vi "Select Ch if asked and Get LR700.vi"(7 "Seconds between samples":dbl=1.0 format="%_4f", 8 "error in (no error)":errorcluster, 10 "Channels to scan (empty - don't use scanner option)":i32[](array[numeric]), 11 "VISA Resource Name":refnum<visa-resource-name>) -> (0 "error out":errorcluster, 2 "Data":dbl[](array[numeric]), 3 "VISA resource name out":refnum<visa-resource-name>)   [LabVIEW 2015]
uses:
  Get LR700 R & X_VISA.vi
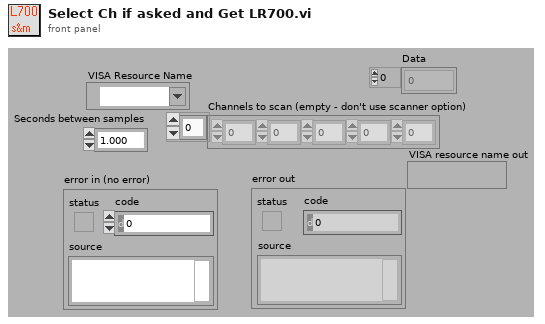
[diagram p1: front panel]
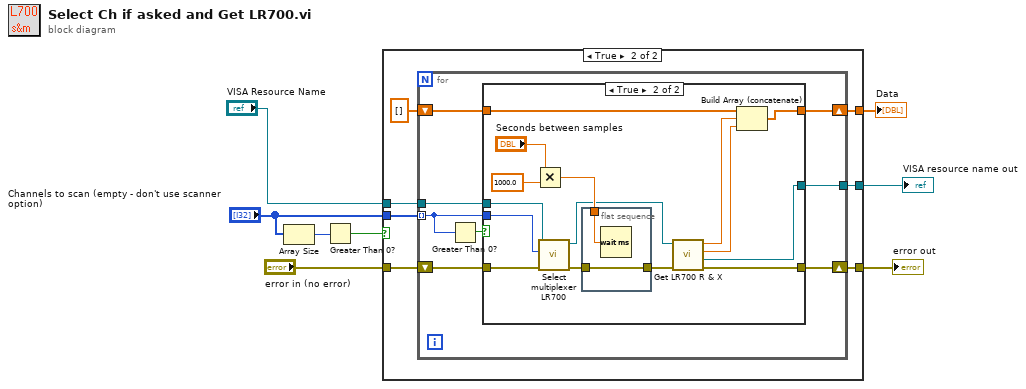
[diagram p0: block diagram]
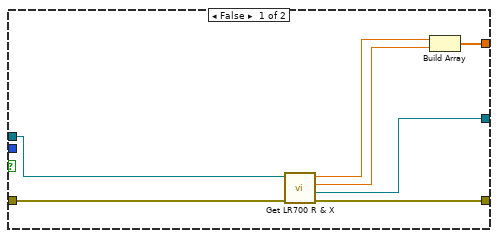
[diagram p2: hidden frame]
diagram:
  n1 = Array Size(array="Channels to scan (empty - don't use scanner option)") -> (size(s)=w8:i32)
  n2 = Greater Than 0?(x=w8) -> (x > 0?=w6:bool)
  n3 = case shown="True" w6 {
    tunnel: "Channels to scan (empty - don't use scanner option)" -> [_ w22]
    tunnel: [w11 w21] -> w5
    tunnel: "error in (no error)" -> [w15 w20]
    tunnel: [w14 w19] -> w3
    tunnel: "VISA Resource Name" -> [w10 w17]
    tunnel: [w9 w16] -> w1
    frame False {
      n4 = call-poly "Get LR700 R & X.vi"("error in (no error)"=w15, "VISA resource name"=w10) -> ("error out"=w14:errorcluster, "VISA resource name out"=w9:refnum<visa-resource-name>, "X"=w12:dbl, "Resistance"=w13:dbl)  [unwired: 2 out]
      n5 = Build Array(w13, w12) -> (w11:dbl[])
    }
    frame True {
      n6 = for {
        tunnel: w22 -> [w30] mode=indexing
        shift-right: [w26] -> w21
        shift-left: dbl[] [] -> [w25]
        shift-right: [w27] -> w19
        shift-left: w20 -> [w29]
        tunnel: w17 -> [w24]
        tunnel: [w23] -> w16
        n7 = Greater Than 0?(x=w30) -> (x > 0?=w28:bool)
        n8 = case shown="True" w28 {
          tunnel: w30 -> [_ w48]
          tunnel: w29 -> [w32 w47]
          tunnel: [w32 w41] -> w27
          tunnel: [w33 w38] -> w26
          tunnel: w25 -> [w33 w37]
          tunnel: w24 -> [w31 w36]
          tunnel: [w31 w34] -> w23
          frame False {
          }
          frame True {
            n9 = Multiply(x="Seconds between samples", y=1000.0) -> (x*y=w42:dbl)
            n10 = call "Select multiplexer LR700.vi"("error in"=w47, "Sensor <01-99>"=w48, "VISA Resource Name"=w36) -> ("error out"=w46:errorcluster, "VISA Resource Name Out"=w35:refnum<visa-resource-name>)  [unwired: 7 out]
            n11 = flat-sequence {
              tunnel: w46 -> [w50]
              tunnel: [w50] -> w45
              tunnel: w42 -> [w49]
              frame #0 {
                n12 = Wait (ms)(milliseconds to wait=w49) -> ()  [unwired: 1 out]
              }
            }
            n13 = call-poly "Get LR700 R & X.vi"("error in (no error)"=w45, "VISA resource name"=w35) -> ("error out"=w41:errorcluster, "VISA resource name out"=w34:refnum<visa-resource-name>, "X"=w39:dbl, "Resistance"=w40:dbl)  [unwired: 2 out]
            n14 = Build Array (concatenate)(w37, w40, w39) -> (w38:dbl[])
          }
        }
      }
    }
  }
  "Data" <- w5
  "error out" <- w3
  "VISA resource name out" <- w1
